vi "Wait_for.vi"(8 "error in (no error)":errorcluster, 10 "Message_command in":T1, 11 "Command Queue":T2) -> (0 "error out":errorcluster, 3 "dup Message_command":T1)   [LabVIEW 2020]
uses:
  Command_Message.ctl
  Command_Queue.ctl
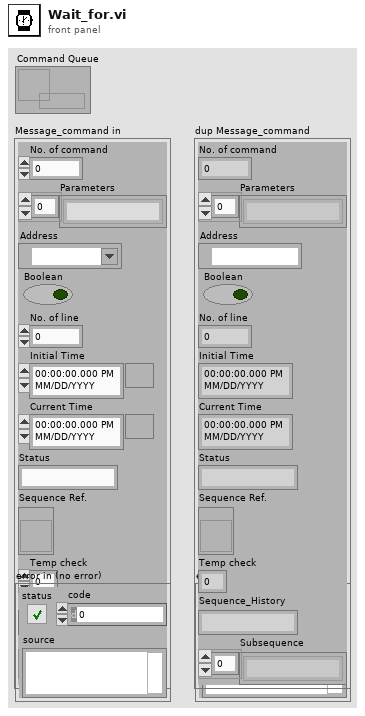
[diagram p1: front panel]
types:
  T1 = typedef "Command_Message.ctl" = cluster{"No. of command":i32, "Parameters":string[], "Address":refnum<visa-resource-name>, "Boolean":bool, "No. of line":i32, "Initial Time":timestamp, "Current Time":timestamp, "Status":string, "Sequence Ref.":refnum<vi>, "Temp check":i32, "Sequence_History":string, "Subsequence":string[]}
  T2 = typedef "Command_Queue.ctl" = refnum<queue>
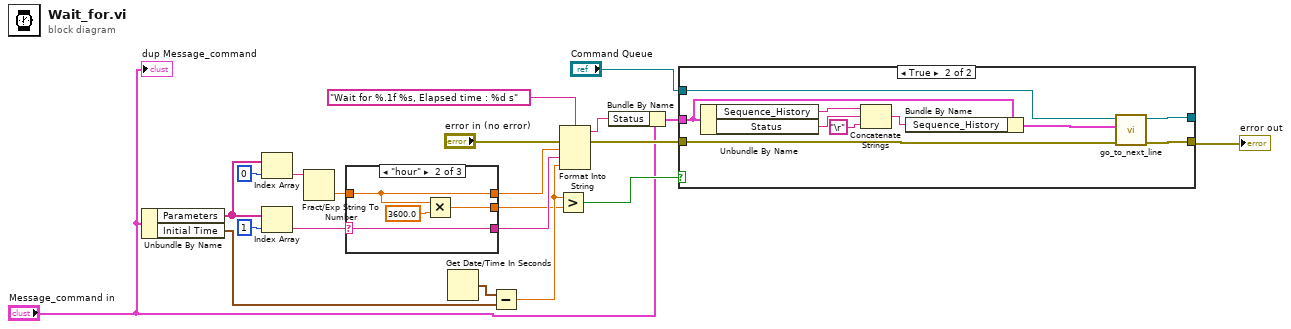
[diagram p0: block diagram]
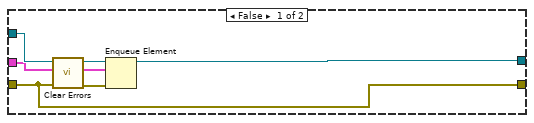
[diagram p2: hidden frame]
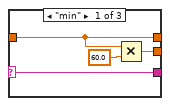
[diagram p3: hidden frame]
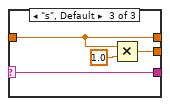
[diagram p4: hidden frame]
diagram:
  n1 = Unbundle By Name("Message_command in") -> ("Parameters"=w15:string[], "Initial Time"=w14:timestamp)
  n2 = Index Array(array=w15, index=0) -> (element=w16:string)
  n3 = Index Array(array=w15, index=1) -> (element=w20:string)
  n4 = Fract/Exp String To Number(string=w16) -> (number=w21:dbl)  [unwired: 3 in, 1 out]
  n5 = case shown="\"hour\"" w20 {
    selector: w20 -> [w22 w26 w30]
    tunnel: w21 -> [w23 w27 w31]
    tunnel: [w24 w28 w32] -> w7
    tunnel: [w22 w26 w30] -> w10
    tunnel: [w23 w27 w31] -> w11
    frame "min" {
      n6 = Multiply(x=w23, y=60.0) -> (x*y=w24:dbl)
    }
    frame "hour" {
      n7 = Multiply(x=w27, y=3600.0) -> (x*y=w28:dbl)
    }
    frame "s", Default {
      n8 = Multiply(x=w31, y=1.0) -> (x*y=w32:dbl)
    }
  }
  n9 = Get Date/Time In Seconds() -> (seconds since 1Jan1904=w17:timestamp)
  n10 = Subtract(x=w17, y=w14) -> (x-y=w8:dbl)
  n11 = Greater?(x=w8, y=w7) -> (0:w6:bool)
  n12 = Format Into String(format string="Wait for %.1f %s, Elapsed time : %d s", error in="error in (no error)", w11, w10, w8) -> (resulting string=w9:string, error out=w5:errorcluster)  [unwired: 1 in]
  n13 = Bundle By Name(cluster="Message_command in", "Status"=w9) -> (w1:T1)
  n14 = case shown="True" w6 {
    tunnel: w5 -> [w34 w48]
    tunnel: "Command Queue" -> [w37 w47]
    tunnel: [w38 w46] -> _
    tunnel: [w34 w45] -> w3
    tunnel: w1 -> [w36 w41]
    frame False {
      n15 = call <vilib>:"Clear Errors.vi"("error in (no error)"=w34) -> ("error out"=w35:errorcluster)  [unwired: 5 in, 1 out]
      n16 = Enqueue Element(queue=w37, element=w36, error in (no error)=w35) -> (queue out=w38:T2)  [unwired: 1 in, 2 out]
    }
    frame True {
      n17 = Unbundle By Name(w41) -> ("Sequence_History"=w44:string, "Status"=w43:string)
      n18 = Concatenate Strings(w44, w43, "\r") -> (w40:string)
      n19 = Bundle By Name(cluster=w41, "Sequence_History"=w40) -> (w39:T1)
      n20 = call "go_to_next_line.vi"("error in (no error)"=w48, "Message_command in"=w39, "Command Queue in"=w47) -> ("error out"=w45:errorcluster, "Command Queue out"=w46:T2)  [unwired: 7 in]
    }
  }
  "error out" <- w3
  "dup Message_command" <- "Message_command in"
